vi "Send_High_Low(SubVI).vi"(9 "error in (no error)":errorcluster, 10 "VISA resource name":refnum<visa-resource-name>, 11 "Set High1 Time":i16) -> (0 "error out":errorcluster, 1 "ASCII string":string[](array[string]), 2 "High1 Time(ns)":dbl, 3 "Digital Outputs":bool[](array[boolean]), 5 "VISA resource name out":refnum<visa-resource-name>, 8 "In Range?":bool)   [LabVIEW 2022 SP3]
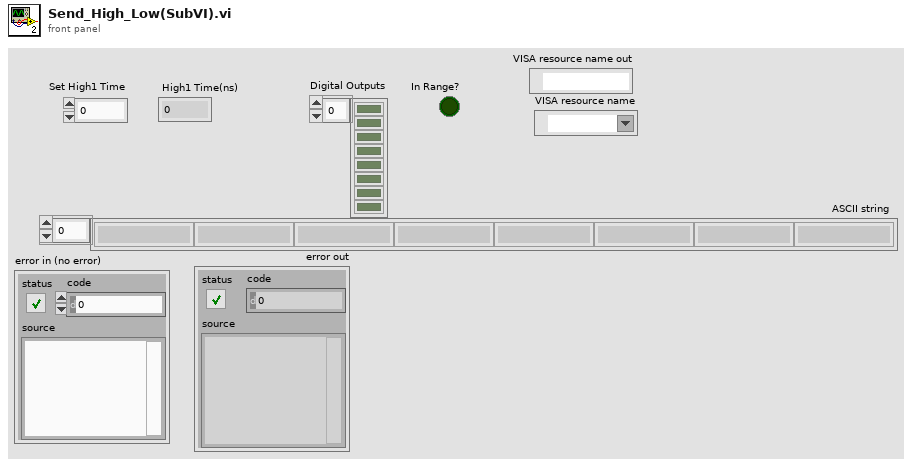
[diagram p1: front panel]
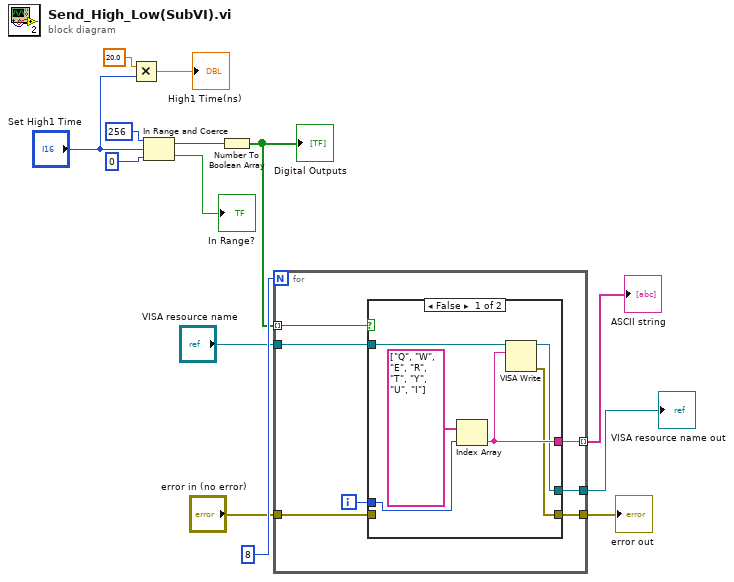
[diagram p0: block diagram]
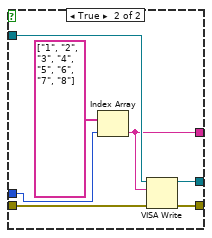
[diagram p2: hidden frame]
diagram:
  n1 = Multiply(x=20.0, y="Set High1 Time") -> (x*y=→"High1 Time(ns)":dbl)
  n2 = In Range and Coerce(upper limit=i16 256, x="Set High1 Time", lower limit=i8 0) -> (coerced(x)=w8:i16, In Range?=→"In Range?":bool)
  n3 = Number To Boolean Array(number=w8) -> (Boolean array=w9:bool[])
  "Digital Outputs" <- w9
  n4 = for {
    N: 8 -> [_]
    tunnel: w9 -> [w21] mode=indexing
    tunnel: [w19] -> w11 mode=indexing
    tunnel: "VISA resource name" -> [w18]
    tunnel: [w17] -> w3
    tunnel: [w16] -> w2
    tunnel: "error in (no error)" -> [w15]
    i -> [w20]
    n5 = case shown="False" w21 {
      tunnel: w20 -> [w27 w33]
      tunnel: [w24 w31] -> w19
      tunnel: w18 -> [w25 w32]
      tunnel: [w23 w30] -> w17
      tunnel: [w22 w29] -> w16
      tunnel: w15 -> [_ w28]
      frame False {
        n6 = Index Array(array=string[] ["Q", "W", "E", "R", "T", "Y", "U", "I"] ("ASCII LOW"), index=w27) -> (element=w24:string)
        n7 = VISA Write(VISA resource name=w25, write buffer=w24) -> (VISA resource name out=w23:refnum<visa-resource-name>, error out=w22:errorcluster)  [unwired: 1 in, 1 out]
      }
      frame True {
        n8 = Index Array(array=string[] ["1", "2", "3", "4", "5", "6", "7", "8"] ("ASCII HIGH"), index=w33) -> (element=w31:string)
        n9 = VISA Write(VISA resource name=w32, write buffer=w31, error in (no error)=w28) -> (VISA resource name out=w30:refnum<visa-resource-name>, error out=w29:errorcluster)  [unwired: 1 out]
      }
    }
  }
  "ASCII string" <- w11
  "VISA resource name out" <- w3
  "error out" <- w2
